vi "Dashboard.vi"() -> ()   [LabVIEW 2026]
uses:
  Control/Ctrl_IndicadoresMainPanel.ctl
  Control/Ctrl_GuiEvent.ctl
  <vilib>/Utility/miscctls.llb/LVPointTypeDef.ctl
panel:
  out "time string":string
  out "Vel_antebrazo":i32 caption="Velocidad"
  out "V_ant":i32 caption="Vueltas"
  out "P_ant":i32 caption="Pasos"
  out "Enc_Antebrazo":i32(knob) caption="Enc. Antebrazo" scale=0.0..196.0
  out "Vel_hombro":i32 caption="Velocidad"
  out "V_hombro":i32 caption="Vueltas"
  out "P_hombro":i32 caption="Pasos"
  out "Enc_Hombro":i32(knob) caption="Enc. Hombro" scale=0.0..400.0
  out "Vel_mun":i32 caption="Velocidad"
  out "V_mun":i32 caption="Vueltas"
  out "P_mun":i32 caption="Pasos"
  out "Enc_Muneca":i32(knob) caption="Enc. Muñeca" scale=0.0..196.0
  out "Vel_codo":i32 caption="Velocidad"
  out "V_cod":i32 caption="Vueltas"
  out "P_cod":i32 caption="Pasos"
  out "Enc_Codo":i32(knob) caption="Enc. Codo" scale=0.0..400.0
  out "Vel_cad":i32 caption="Velocidad"
  out "V_cad":i32 caption="Vueltas"
  out "P_cad":i32 caption="Pasos"
  out "Enc_Cadera":i32(knob) caption="Enc. Cadera" scale=0.0..400.0
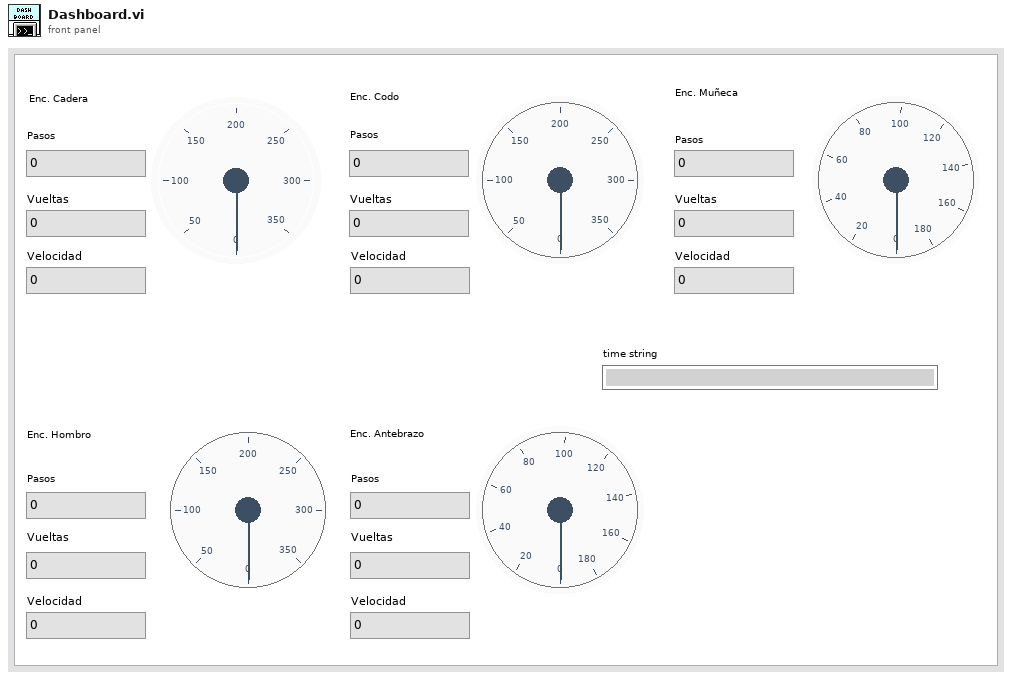
[diagram p1: front panel]
types:
  T1 = typedef "Ctrl_GuiEvent.ctl" = enum16{"Set Ref", "Update Enc", "Stop", "Get Ref"}
  T2 = typedef "Ctrl_IndicadoresMainPanel.ctl" = cluster{"status_serial":refnum<vi>, "Vel_cad":refnum<vi>, "Vel_antebrazo":refnum<vi>, "Vel_hombro":refnum<vi>, "Vel_mun":refnum<vi>, "Vel_codo":refnum<vi>, "P_mun":refnum<vi>, "P_ant":refnum<vi>, "P_cod":refnum<vi>, "P_hombro":refnum<vi>, "P_cad":refnum<vi>, "Enc_Antebrazo":refnum<vi>, "Enc_Codo":refnum<vi>, "Enc_Muneca":refnum<vi>, "Enc_Hombro":refnum<vi>, "Enc_Cadera":refnum<vi>, "V_mun":refnum<vi>, "V_ant":refnum<vi>, "V_hombro":refnum<vi>, "V_cod":refnum<vi>, "V_cad":refnum<vi>, "LS_Cadera":refnum<vi>, "LS_Hombro":refnum<vi>, "LS_Antebrazo":refnum<vi>, "LS_Codo":refnum<vi>, "Freno_hombro":refnum<vi>, "Freno_codo":refnum<vi>}
  T3 = typedef "LVPointTypeDef.ctl" = cluster{"Horizontal":i16, "Vertical":i16}
  T4 = typedef "Ctrl_Array_Enc_Out.ctl" = T5[]
  T5 = typedef "Ctr_Enc_Values.ctl" = cluster{"Datos6_Motores":T6, "Errores":T8, "new_data?":bool}
  T6 = typedef "Ctrl_datos6motores_final.ctl" = cluster{"M_cadera":T7, "M_hombro":T7, "M_codo":T7, "M_antebrazo":T7, "M_muneca":T7, "M_gripper":T7}
  T7 = typedef "Ctrl_Motores_Valores.ctl" = cluster{"Pasos":i32, "Vueltas":i16, "Velocidad":dbl, "Reserva1":u8, "Reserva2":u8}
  T8 = typedef "Ctrl_Errores.ctl" = cluster{"Contador_correcto":u32, "Contador_errores":u32, "Edo_conex":u32}
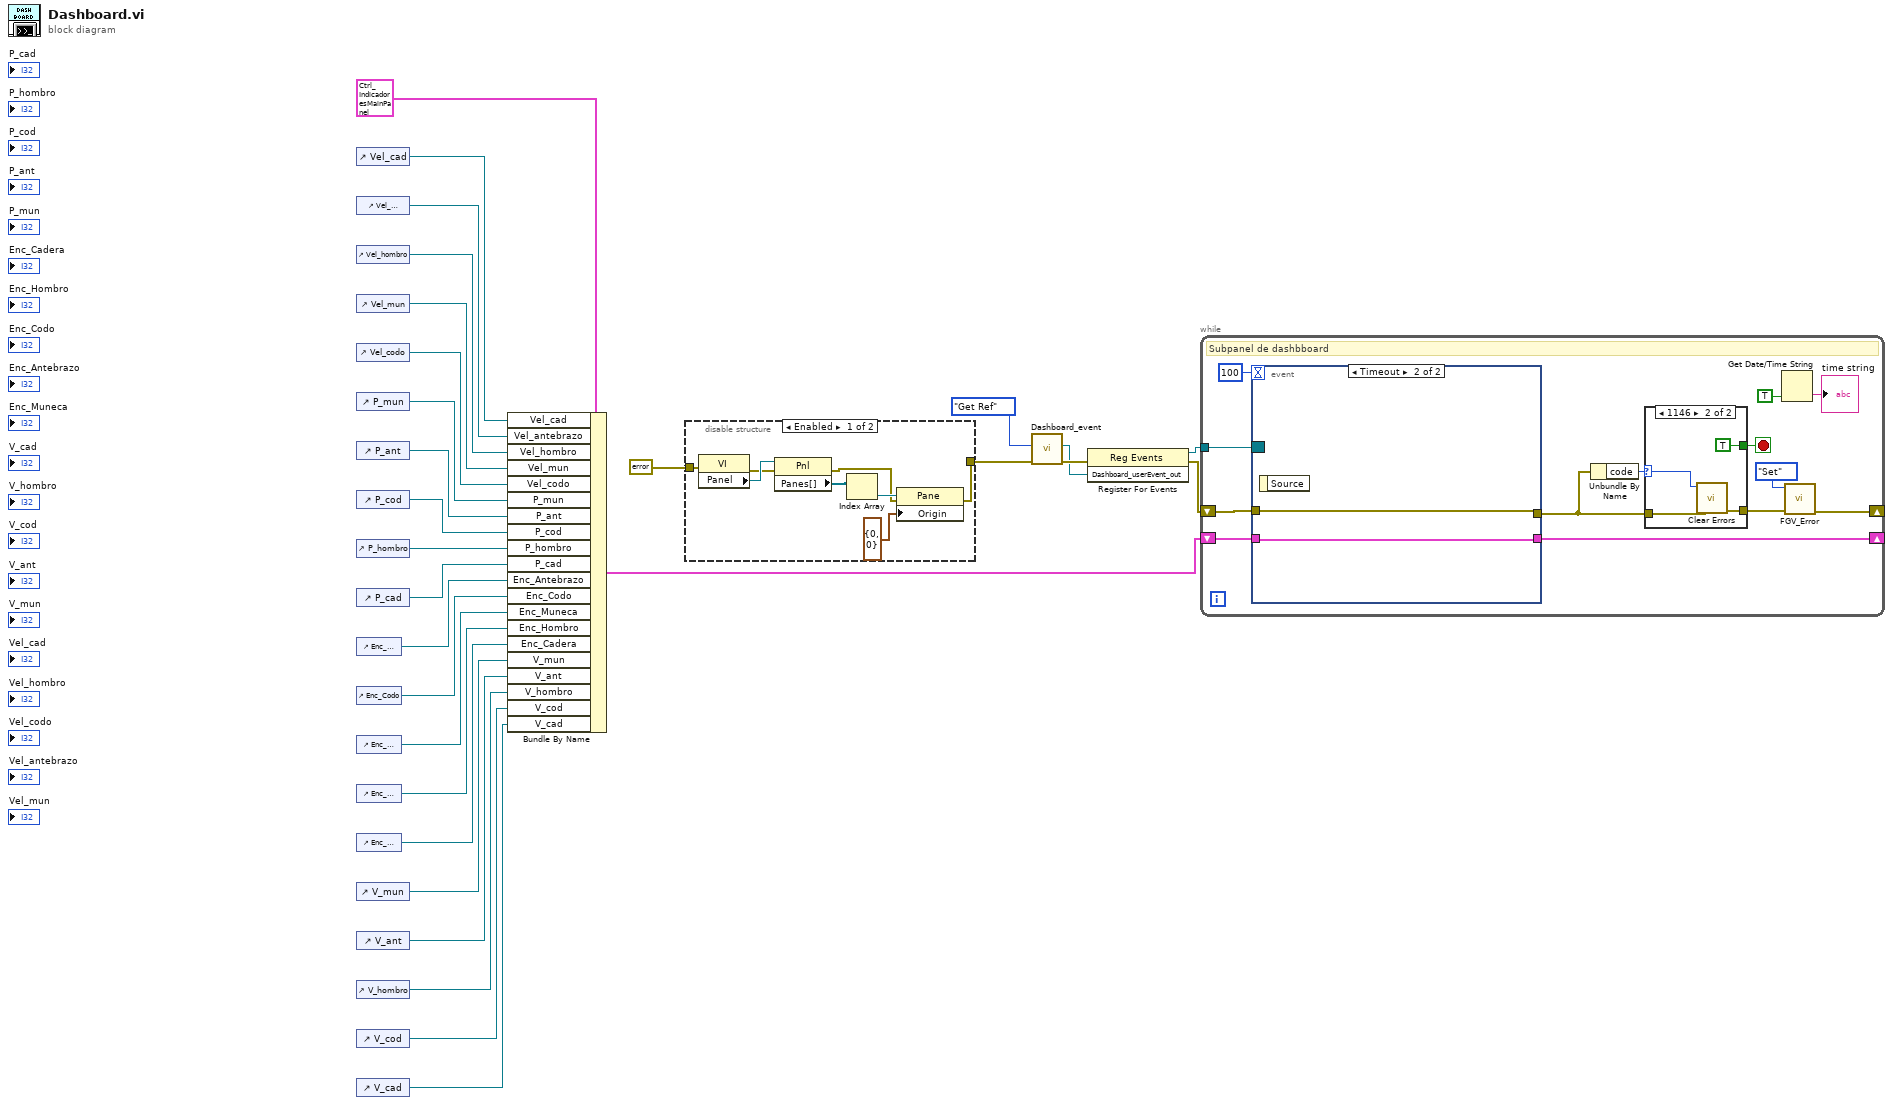
[diagram p0: block diagram]
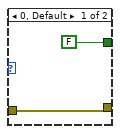
[diagram p3: hidden frame]
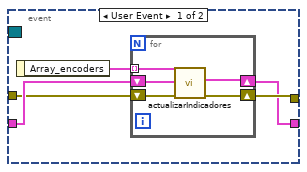
[diagram p4: hidden frame]
diagram:
  n1 = control-ref of="Vel_cad"() -> (w13:refnum<vi>)
  n2 = control-ref of="Vel_antebrazo"() -> (w10:refnum<vi>)
  n3 = control-ref of="Vel_hombro"() -> (w12:refnum<vi>)
  n4 = control-ref of="Vel_mun"() -> (w9:refnum<vi>)
  n5 = control-ref of="Vel_codo"() -> (w11:refnum<vi>)
  n6 = control-ref of="P_mun"() -> (w25:refnum<vi>)
  n7 = control-ref of="P_ant"() -> (w26:refnum<vi>)
  n8 = control-ref of="P_cod"() -> (w27:refnum<vi>)
  n9 = control-ref of="P_hombro"() -> (w28:refnum<vi>)
  n10 = control-ref of="P_cad"() -> (w29:refnum<vi>)
  n11 = control-ref of="Enc_Antebrazo"() -> (w21:refnum<vi>)
  n12 = control-ref of="Enc_Codo"() -> (w22:refnum<vi>)
  n13 = control-ref of="Enc_Muneca"() -> (w20:refnum<vi>)
  n14 = control-ref of="Enc_Hombro"() -> (w23:refnum<vi>)
  n15 = control-ref of="Enc_Cadera"() -> (w24:refnum<vi>)
  n16 = control-ref of="V_mun"() -> (w15:refnum<vi>)
  n17 = control-ref of="V_ant"() -> (w16:refnum<vi>)
  n18 = control-ref of="V_hombro"() -> (w18:refnum<vi>)
  n19 = control-ref of="V_cod"() -> (w17:refnum<vi>)
  n20 = control-ref of="V_cad"() -> (w19:refnum<vi>)
  n21 = Bundle By Name(cluster=T2 {"status_serial"=refnum, "Vel_cad"=refnum, "Vel_antebrazo"=refnum, "Vel_hombro"=refnum, "Vel_mun"=refnum, "Vel_codo"=refnum, "P_mun"=refnum, "P_ant"=refnum, "P_cod"=refnum, "P_hombro"=refnum, "P_cad"=refnum, "Enc_Antebrazo"=refnum, "Enc_Codo"=refnum, "Enc_Muneca"=refnum, "Enc_Hombro"=refnum, "Enc_Cadera"=refnum, "V_mun"=refnum, "V_ant"=refnum, "V_hombro"=refnum, "V_cod"=refnum, "V_cad"=refnum, "LS_Cadera"=refnum, "LS_Hombro"=refnum, "LS_Antebrazo"=refnum, "LS_Codo"=refnum, "Freno_hombro"=refnum, "Freno_codo"=refnum} ("output cluster"), "Vel_cad"=w13, "Vel_antebrazo"=w10, "Vel_hombro"=w12, "Vel_mun"=w9, "Vel_codo"=w11, "P_mun"=w25, "P_ant"=w26, "P_cod"=w27, "P_hombro"=w28, "P_cad"=w29, "Enc_Antebrazo"=w21, "Enc_Codo"=w22, "Enc_Muneca"=w20, "Enc_Hombro"=w23, "Enc_Cadera"=w24, "V_mun"=w15, "V_ant"=w16, "V_hombro"=w18, "V_cod"=w17, "V_cad"=w19) -> (w8:T2)
  n22 = disable-structure shown="Enabled" {
    disable-tunnel: errorcluster {"status"=FALSE, "code"=0, "source"=""} ("error out") -> [w33 w38]
    disable-tunnel: [w31 w38] -> w2
    frame Enabled {
      n23 = property class="VI"(error in=w33) -> (error out=w36:errorcluster, "Panel"=w37:refnum<vi>)  [unwired: 1 in, 1 out]
      n24 = property class="Pnl"(reference=w37, error in=w36) -> (error out=w32:errorcluster, "Panes[]"=w35:refnum<vi>[])  [unwired: 1 out]
      n25 = Index Array(array=w35) -> (element=w34:refnum<vi>)  [unwired: 1 in]
      n26 = property class="Pane"(reference=w34, error in=w32, "Origin"=T3 {"Horizontal"=0, "Vertical"=0}) -> (error out=w31:errorcluster)  [unwired: 1 out]
    }
    frame Disabled {
    }
  }
  n27 = call "Dashboard_event.vi"("error in"=w2, "Estado"=Ctrl_GuiEvent."Get Ref") -> ("error out"=w7:errorcluster, "Dashboard_userEvent_out"=w6:refnum<user-event>)  [unwired: 8 in]
  n28 = register-events(error in=w7, w6) -> (reference out=w4:refnum<event-registration>, error out=w5:errorcluster)  [unwired: 1 in]
  n29 = while {
    shift-right: [w46] -> _
    shift-left: w8 -> [w49]
    shift-right: [w48] -> _
    shift-left: w5 -> [w50]
    tunnel: w4 -> [w51]
    stop <- w42 stop-if-true
    # "Subpanel de dashbboard"
    n30 = event shown="[1] Timeout" {
      selector: w51 -> [_ _]
      dyn-events: _ -> [_ _]
      timeout: 100 -> [_ _]
      tunnel: w50 -> [w61 w69]
      tunnel: w49 -> [w62 w68]
      tunnel: [w60 w69] -> w44
      tunnel: [w58 w68] -> w46
      event User Event {
        n31 = event-data() -> ("Array_encoders"=w59:T4)  [unwired: 1 in]
        n32 = for {
          shift-right: [w66] -> w60
          shift-left: w61 -> [w67]
          shift-right: [w64] -> w58
          shift-left: w62 -> [w65]
          tunnel: w59 -> [w63] mode=indexing
          n33 = call "actualizarIndicadores.vi"("error in (no error) 2"=w67, "indicator_cluster_in"=w65, "Enc_values_in"=w63) -> ("error out"=w66:errorcluster, "indicator_cluster_out"=w64:T2)  [unwired: 6 in, 1 out]
        }
      }
      event Timeout {
        n34 = event-data() -> ()  [unwired: 1 in, 1 out]
      }
    }
    n35 = Unbundle By Name(w44) -> ("code"=w45:i32)
    n36 = case shown="1146" w45 {
      selector: w45 -> [_ w56]
      tunnel: w44 -> [w53 w57]
      tunnel: [w53 w55] -> w43
      tunnel: [FALSE TRUE] -> w42
      frame 0, Default {
      }
      frame 1146 {
        n37 = call <vilib>:"Clear Errors.vi"("error in (no error)"=w57, "specific error code to clear (0: all)"=w56) -> ("error out"=w55:errorcluster)  [unwired: 4 in, 1 out]
      }
    }
    n38 = Get Date/Time String(want seconds? (F)=TRUE) -> (time string=→"time string":string)  [unwired: 2 in, 1 out]
    n39 = call "FGV_Error.vi"("error_in_loop"=w43, "Estado"=enum16{"Set", "Get"}."Set") -> ("error out"=w48:errorcluster)  [unwired: 9 in]
  }
